vi "Overlay_test.vi"(7 "Out of bounds coord":cluster{"X":sgl, "Y":sgl}[](array[cluster]), 8 "error in":errorcluster, 9 "Overlay Info":T2, 10 "Type":string, 11 "Image":T1) -> (0 "error out":errorcluster, 3 "WithinImage?":bool)   [LabVIEW 2015]
uses:
  <vilib>/vision/Image Controls.llb/IMAQ Image.ctl
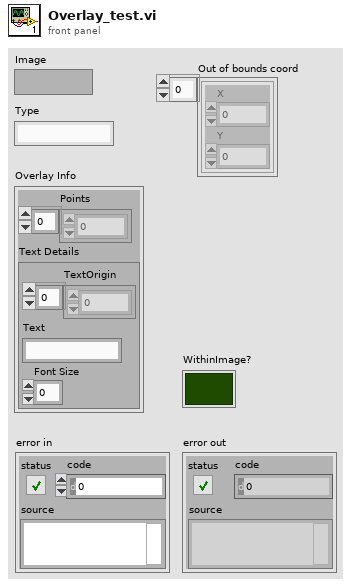
[diagram p1: front panel]
types:
  T1 = typedef "IMAQ Image.ctl" = refnum<image>
  T2 = cluster{"Points":dbl[], "Text Details":cluster{"TextOrigin":dbl[], "Text":string, "Font Size":u32}}
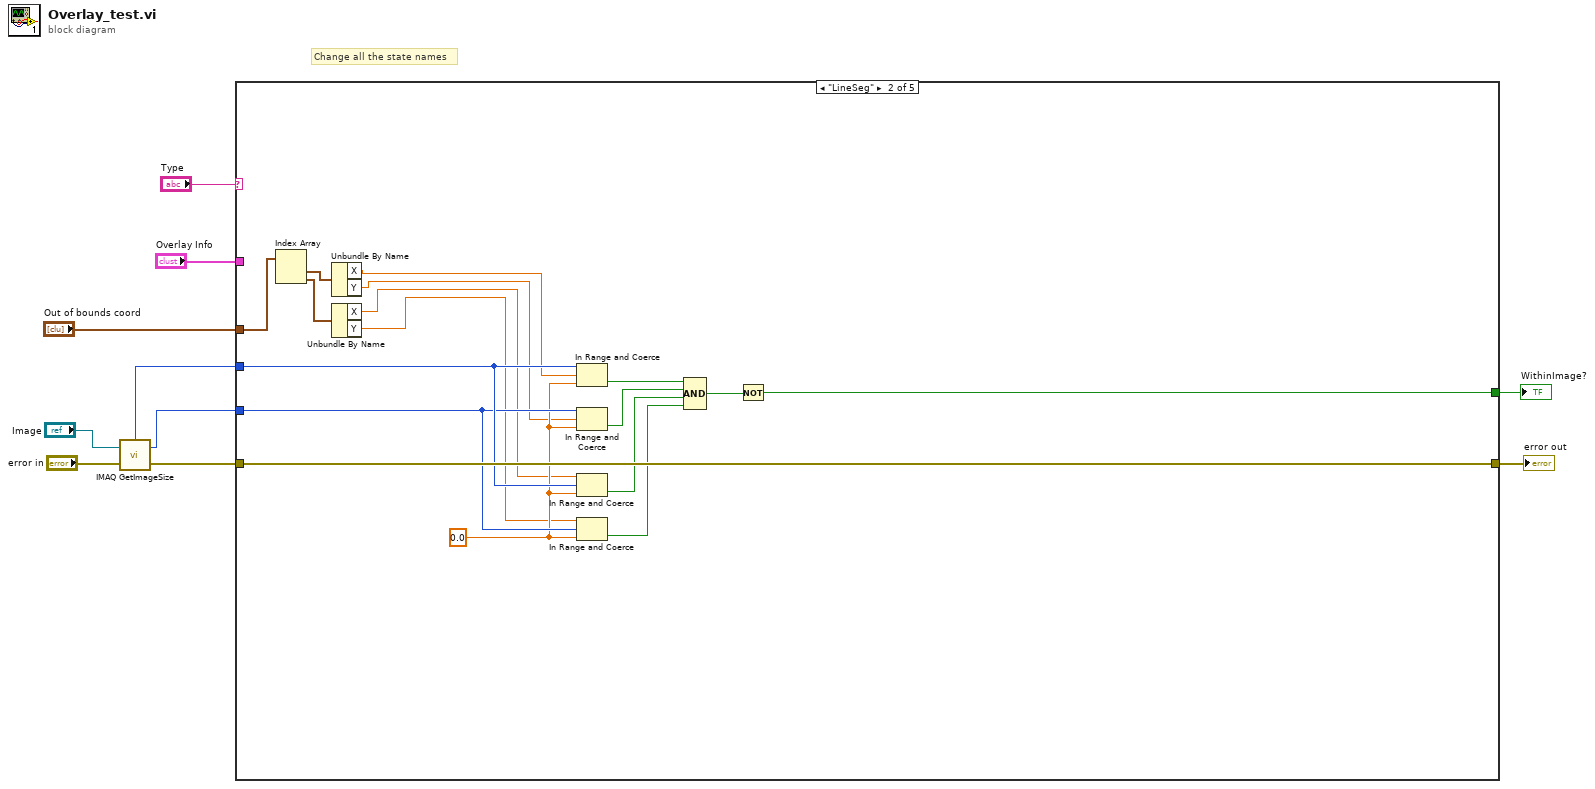
[diagram p0: block diagram]
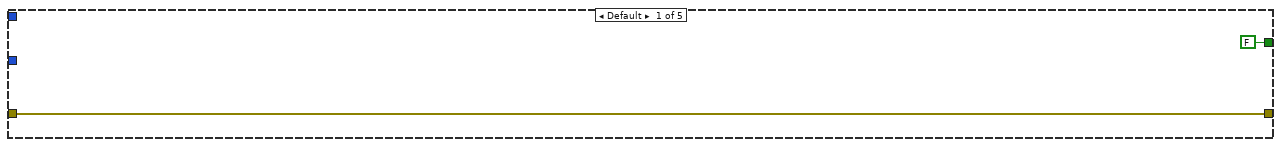
[diagram p2: hidden frame]
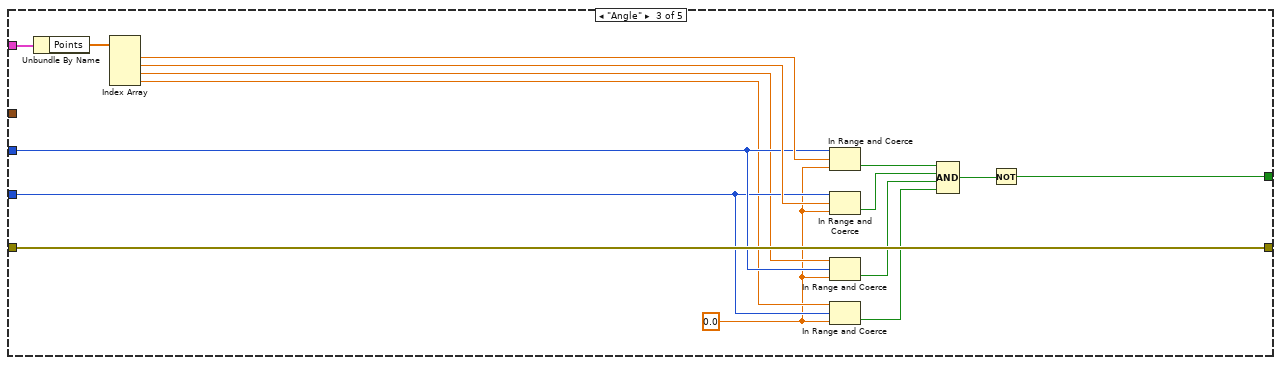
[diagram p3: hidden frame]
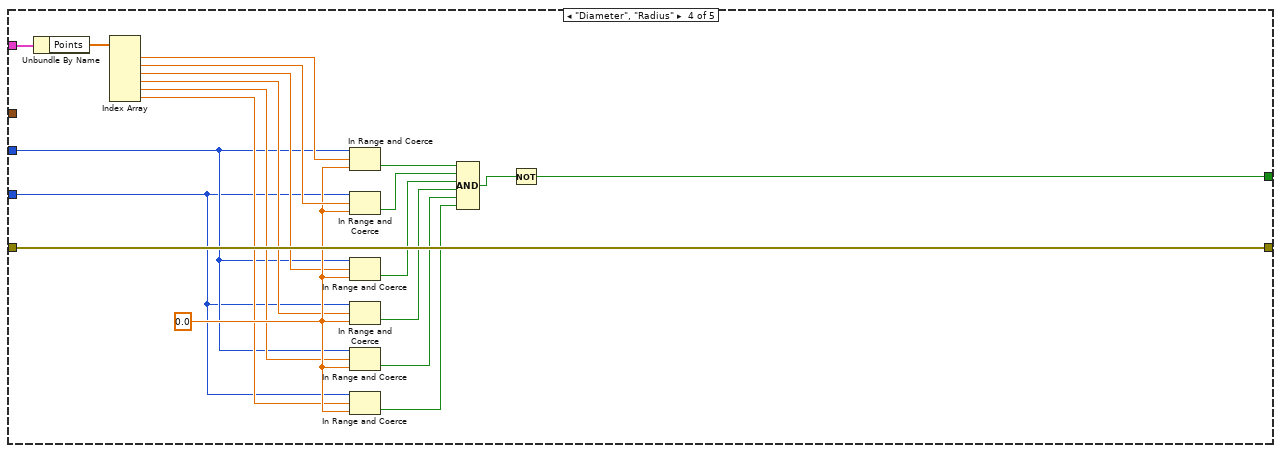
[diagram p4: hidden frame]
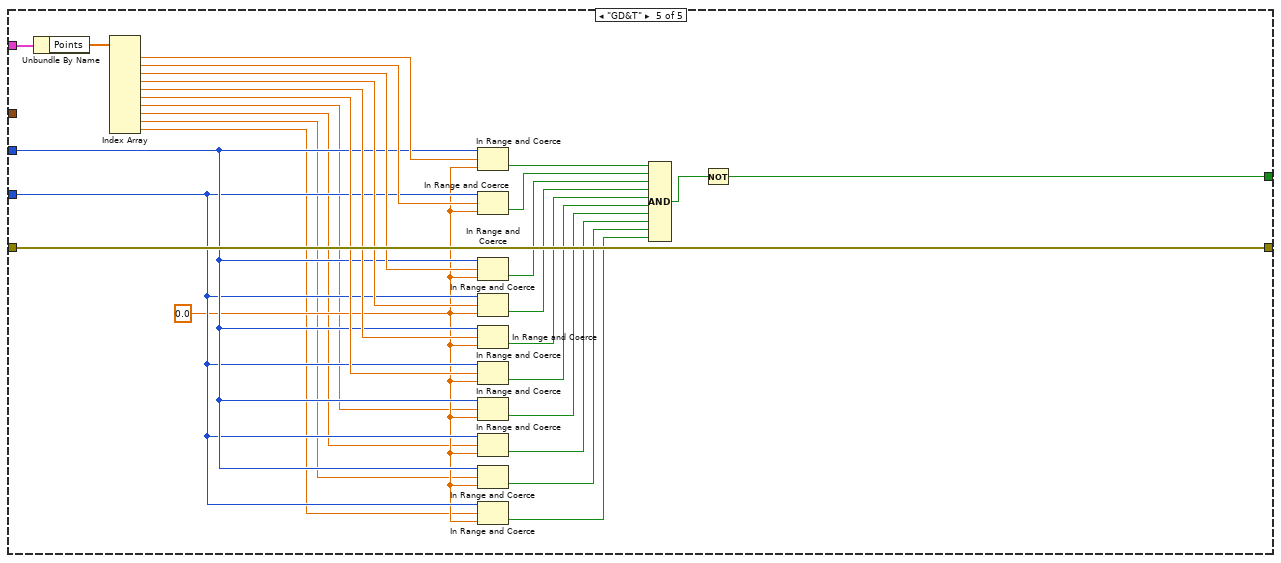
[diagram p5: hidden frame]
diagram:
  # "Change all the state names"
  n1 = call "IMAQ GetImageSize"("Image"="Image", "error in (no error)"="error in") -> ("Y Resolution"=w8:i32, "X Resolution"=w9:i32, "error out"=w7:errorcluster)  [unwired: 2 in]
  n2 = case shown="\"LineSeg\"" "Type" {
    tunnel: w9 -> [_ w28 w40 w49 w76]
    tunnel: w8 -> [_ w27 w39 w48 w75]
    tunnel: w7 -> [w12 w29 w43 w63 w91]
    tunnel: "Overlay Info" -> [_ _ w45 w65 w93]
    tunnel: [w12 w29 w43 w63 w91] -> w5
    tunnel: [FALSE w20 w30 w55 w83] -> w4
    tunnel: "Out of bounds coord" -> [_ w19 _ _ _]
    frame Default {
    }
    frame "LineSeg" {
      w26 = 0.0
      n3 = Index Array(array=w19) -> (element #1=w18:cluster{"X":sgl, "Y":sgl}, element #2=w17:cluster{"X":sgl, "Y":sgl})  [unwired: 2 in]
      n4 = Unbundle By Name(w18) -> ("X"=w16:sgl, "Y"=w15:sgl)
      n5 = Unbundle By Name(w17) -> ("X"=w14:sgl, "Y"=w13:sgl)
      n6 = In Range and Coerce(upper limit=w28, x=w16, lower limit=w26) -> (In Range?=w25:bool)  [unwired: 1 out]
      n7 = In Range and Coerce(upper limit=w27, x=w15, lower limit=w26) -> (In Range?=w24:bool)  [unwired: 1 out]
      n8 = In Range and Coerce(upper limit=w14, x=w28, lower limit=w26) -> (In Range?=w23:bool)  [unwired: 1 out]
      n9 = In Range and Coerce(upper limit=w13, x=w27, lower limit=w26) -> (In Range?=w22:bool)  [unwired: 1 out]
      n10 = Compound Arithmetic op=AND(w25, w24, w23, w22) -> (w21:bool)
      n11 = Not(x=w21) -> (.not. x?=w20:bool)
    }
    frame "Angle" {
      w36 = 0.0
      n12 = Unbundle By Name(w45) -> ("Points"=w44:dbl[])
      n13 = Index Array(array=w44) -> (element #1=w42:dbl, element #2=w41:dbl, element #3=w38:dbl, element #4=w37:dbl)  [unwired: 4 in]
      n14 = In Range and Coerce(upper limit=w40, x=w42, lower limit=w36) -> (In Range?=w35:bool)  [unwired: 1 out]
      n15 = In Range and Coerce(upper limit=w39, x=w41, lower limit=w36) -> (In Range?=w34:bool)  [unwired: 1 out]
      n16 = In Range and Coerce(upper limit=w38, x=w40, lower limit=w36) -> (In Range?=w33:bool)  [unwired: 1 out]
      n17 = In Range and Coerce(upper limit=w37, x=w39, lower limit=w36) -> (In Range?=w32:bool)  [unwired: 1 out]
      n18 = Compound Arithmetic op=AND(w35, w34, w33, w32) -> (w31:bool)
      n19 = Not(x=w31) -> (.not. x?=w30:bool)
    }
    frame "Diameter", "Radius" {
      w54 = 0.0
      n20 = Unbundle By Name(w65) -> ("Points"=w64:dbl[])
      n21 = Index Array(array=w64) -> (element #1=w62:dbl, element #2=w61:dbl, element #3=w50:dbl, element #4=w51:dbl, element #5=w53:dbl, element #6=w52:dbl)  [unwired: 6 in]
      n22 = In Range and Coerce(upper limit=w49, x=w62, lower limit=w54) -> (In Range?=w60:bool)  [unwired: 1 out]
      n23 = In Range and Coerce(upper limit=w48, x=w61, lower limit=w54) -> (In Range?=w59:bool)  [unwired: 1 out]
      n24 = In Range and Coerce(upper limit=w49, x=w50, lower limit=w54) -> (In Range?=w58:bool)  [unwired: 1 out]
      n25 = In Range and Coerce(upper limit=w48, x=w51, lower limit=w54) -> (In Range?=w57:bool)  [unwired: 1 out]
      n26 = In Range and Coerce(upper limit=w49, x=w53, lower limit=w54) -> (In Range?=w47:bool)  [unwired: 1 out]
      n27 = In Range and Coerce(upper limit=w48, x=w52, lower limit=w54) -> (In Range?=w46:bool)  [unwired: 1 out]
      n28 = Compound Arithmetic op=AND(w60, w59, w58, w57, w47, w46) -> (w56:bool)
      n29 = Not(x=w56) -> (.not. x?=w55:bool)
    }
    frame "GD&T" {
      w74 = 0.0
      n30 = Unbundle By Name(w93) -> ("Points"=w92:dbl[])
      n31 = Index Array(array=w92) -> (element #1=w90:dbl, element #2=w89:dbl, element #3=w79:dbl, element #4=w80:dbl, element #5=w82:dbl, element #6=w81:dbl, element #7=w73:dbl, element #8=w72:dbl, element #9=w71:dbl, element #10=w70:dbl)  [unwired: 10 in]
      n32 = In Range and Coerce(upper limit=w76, x=w90, lower limit=w74) -> (In Range?=w88:bool)  [unwired: 1 out]
      n33 = In Range and Coerce(upper limit=w75, x=w89, lower limit=w74) -> (In Range?=w87:bool)  [unwired: 1 out]
      n34 = In Range and Coerce(upper limit=w76, x=w79, lower limit=w74) -> (In Range?=w86:bool)  [unwired: 1 out]
      n35 = In Range and Coerce(upper limit=w75, x=w80, lower limit=w74) -> (In Range?=w85:bool)  [unwired: 1 out]
      n36 = In Range and Coerce(upper limit=w76, x=w82, lower limit=w74) -> (In Range?=w78:bool)  [unwired: 1 out]
      n37 = In Range and Coerce(upper limit=w75, x=w81, lower limit=w74) -> (In Range?=w77:bool)  [unwired: 1 out]
      n38 = In Range and Coerce(upper limit=w76, x=w73, lower limit=w74) -> (In Range?=w69:bool)  [unwired: 1 out]
      n39 = In Range and Coerce(upper limit=w75, x=w72, lower limit=w74) -> (In Range?=w68:bool)  [unwired: 1 out]
      n40 = In Range and Coerce(upper limit=w76, x=w71, lower limit=w74) -> (In Range?=w67:bool)  [unwired: 1 out]
      n41 = In Range and Coerce(upper limit=w75, x=w70, lower limit=w74) -> (In Range?=w66:bool)  [unwired: 1 out]
      n42 = Compound Arithmetic op=AND(w88, w87, w86, w85, w78, w77, w69, w68, w67, w66) -> (w84:bool)
      n43 = Not(x=w84) -> (.not. x?=w83:bool)
    }
  }
  "error out" <- w5
  "WithinImage?" <- w4
